vi "RGB_panicle_processing.vi"() -> ()   [LabVIEW 2019]
uses:
  <vilib>/Utility/file.llb/Read Delimited Spreadsheet (string).vi
  <vilib>/Utility/file.llb/Write Delimited Spreadsheet (string).vi
  <vilib>/vision/NI_Vision_Development_Module.lvlib
  <vilib>/Analysis/NI_AALBase.lvlib
  imFillRemove_vs2019/x64/Release/imFillRemove_vs2019.dll
panel:
  out "mean":dbl format="%0.2f"
  out "sum":dbl
  in  "图片存储":path=path "I:/rice_panicle/org/segment"
  out "Combine Image 7":T1(plugin-control)
  in  "图片来源":path=path "I:/rice_panicle/org/barcode1.txt"
  out "standard deviation 9":dbl format="%0.2f"
  out "mean 9":dbl format="%0.2f"
  out "standard deviation 8":dbl format="%0.2f"
  out "mean 8":dbl format="%0.2f"
  out "standard deviation 7":dbl format="%0.2f"
  out "mean 7":dbl format="%0.2f"
  out "standard deviation 6":dbl format="%0.2f"
  out "mean 6":dbl format="%0.2f"
  out "standard deviation 5":dbl format="%0.2f"
  out "mean 5":dbl format="%0.2f"
  out "Circularity":dbl[](array[numeric])
  out "Equivalent ellipse":dbl[](array[numeric])
  out "AR":dbl[](array[numeric])
  out "Perimeter":dbl[](array[numeric])
  out "Area":dbl[](array[numeric])
  out "耗时":u32
  out "属于某个角度下图像":T1(plugin-control)
  out "粒长":dbl[](array[numeric])
  out "粒宽":dbl[](array[numeric])
  out "长宽比":dbl[](array[numeric])
  out "mean 2":dbl format="%0.2f"
  out "standard deviation 2":dbl format="%0.2f"
  out "mean 3":dbl format="%0.2f"
  out "standard deviation 3":dbl format="%0.2f"
  out "mean 4":dbl format="%0.2f"
  out "standard deviation 4":dbl format="%0.2f"
  in  "数据存储":path=path "I:/rice_panicle/org/data.txt"
  out "估算粒子数目":dbl
  out "Combine Image 6":T1(plugin-control)
  out "selected path":path
  out "Combine Image 5":T1(plugin-control)
  out "Combine Image 4":T1(plugin-control)
  out "Combine Image 3":T1(plugin-control)
  out "Combine Image 2":T1(plugin-control)
  out "Combine Image":T1(plugin-control)
  in  "Range Upper Value":dbl=1200.0
  in  "Range Lower Value":dbl=600.0
  out "Number of Particles 2":i32
  in  "Removeareathreshold 3":i32=600
  in  "Range":cluster{"Lower value":sgl, "Upper value":sgl}={"Lower value"=0.0, "Upper value"=128.0}
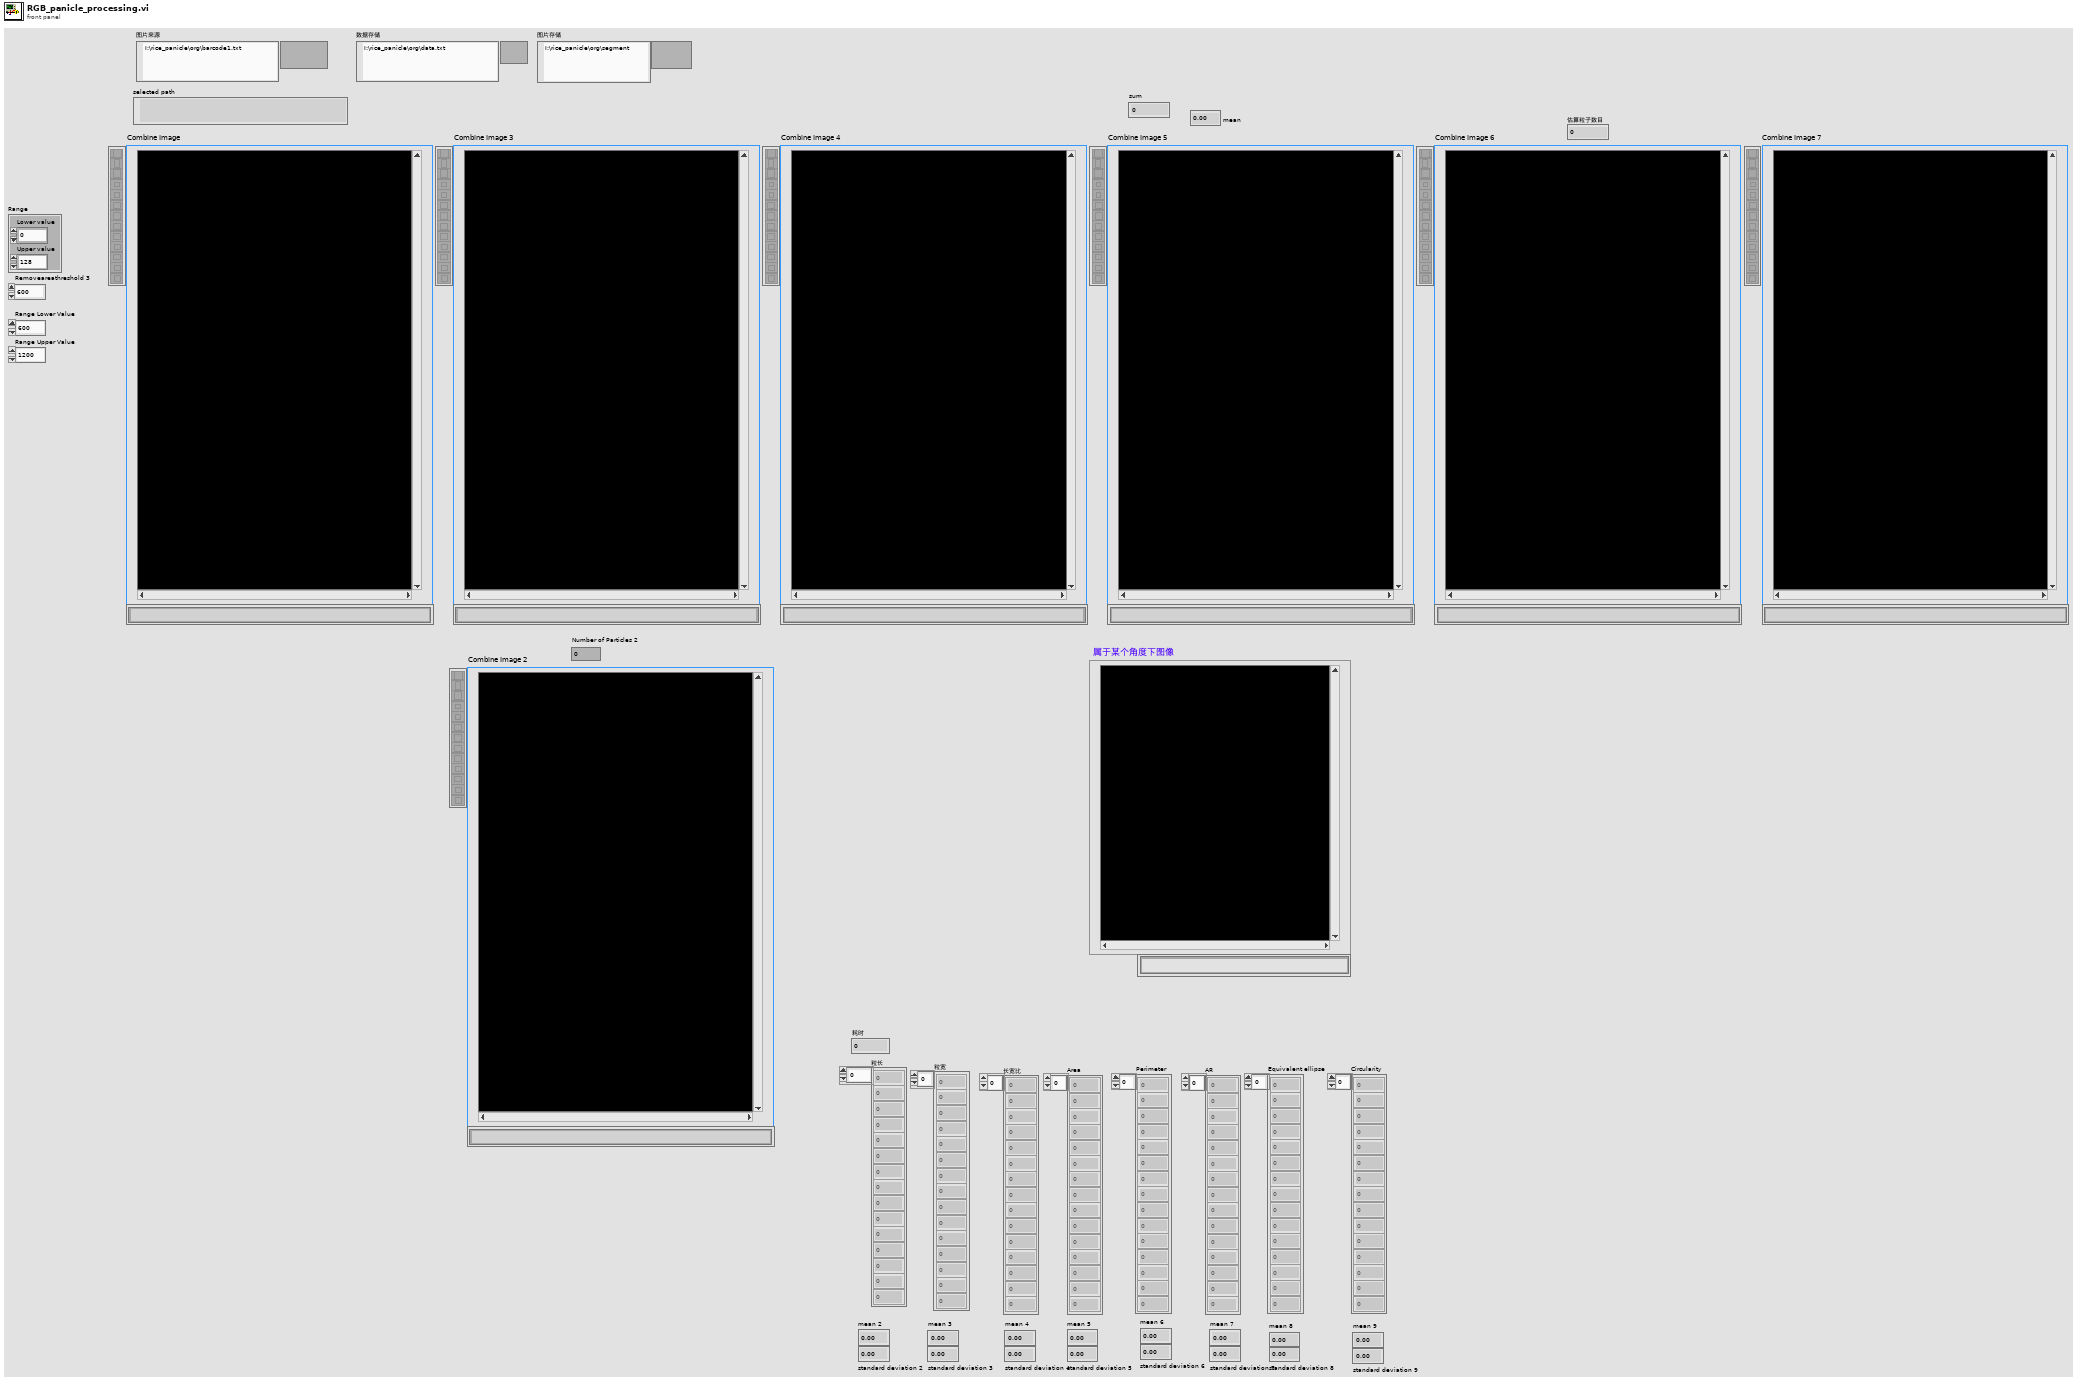
[diagram p1: front panel]
types:
  T1 = typedef "IMAQ Image.ctl" = refnum<image>
  T2 = typedef "Particle Parameters" = i32
  T3 = cluster{"Measurement Parameter":T2, "Range Lower Value":dbl, "Range Upper Value":dbl, "Range":bool, "Measurement Type":bool}
  T4 = enum32{"AutoM", "Close", "Dilate", "Erode", "Gradient", "Gradient out", "Gradient in", "Hit miss", "Open", "PClose", "POpen", "Thick", "Thin"}
  T5 = typedef "Image Type" = u32
  T6 = cluster{"Measurement Parameter":T2, "Range Lower Value":dbl, "Range Upper Value":dbl, "Range":bool, "Measurement Type":bool}[]
  T7 = cluster{"Measurement Parameter":T2, dbl, dbl, "Range":bool, "Measurement Type":bool}
  T8 = cluster{"Measurement Parameter":T2, dbl, dbl, "Range":bool, "Measurement Type":bool}[]
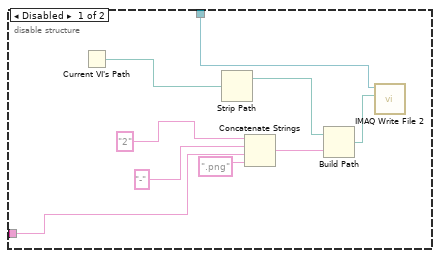
[diagram p2: hidden frame]
diagram:
  n1 = call-poly <vilib>:"Read Delimited Spreadsheet.vi"("file path (dialog if empty)"="图片来源") -> ("all rows"=w4:string[][])  [unwired: 9 in, 5 out]
  n2 = Index Array(array=w4, index (col)=0 ("disabled index (col)")) -> (element=w2:string[])  [unwired: 1 in]
  n3 = for {
    N: 1516 -> [_]
    tunnel: w2 -> [w46] mode=indexing
    w15 = T5 0 items=["Grayscale (U8)", "Grayscale (I16)", "Grayscale (SGL)", "Complex (CSG)", "RGB (U32)", "HSL (U32)", "RGB (U64)", "Grayscale (U16)"] ("Image Type")
    w22 = T5 0 items=["Grayscale (U8)", "Grayscale (I16)", "Grayscale (SGL)", "Complex (CSG)", "RGB (U32)", "HSL (U32)", "RGB (U64)", "Grayscale (U16)"] ("Image Type")
    w34 = T5 4 items=["Grayscale (U8)", "Grayscale (I16)", "Grayscale (SGL)", "Complex (CSG)", "RGB (U32)", "HSL (U32)", "RGB (U64)", "Grayscale (U16)"] ("Image Type")
    w79 = T2[] [35, 19, 32, 50, 55] items=["Center of Mass X", "Center of Mass Y", "First Pixel X", "First Pixel Y", "Bounding Rect Left", "Bounding Rect Top", "Bounding Rect Right", "Bounding Rect Bottom", "Max Feret Diameter Start X", "Max Feret Diameter Start Y", "Max Feret Diameter End X", "Max Feret Diameter End Y", "Max Horiz. Segment Length Left", "Max Horiz. Segment Length Right", "Max Horiz. Segment Length Row", "-", "Bounding Rect Width", "Bounding Rect Height", "Bounding Rect Diagonal", "Perimeter", "Convex Hull Perimeter", "Holes' Perimeter", "Max Feret Diameter", "Equivalent Ellipse Major Axis", "Equivalent Ellipse Minor Axis", "Equivalent Ellipse Minor Axis (Feret)", "Equivalent Rect Long Side", "Equivalent Rect Short Side", "Equivalent Rect Diagonal", "Equivalent Rect Short Side (Feret)", "Average Horiz. Segment Length", "Average Vert. Segment Length", "Hydraulic Radius", "Waddel Disk Diameter", "-", "Area", "Holes' Area", "Particle & Holes' Area", "Convex Hull Area", "Image Area", "-", "Number of Holes", "Number of Horiz. Segments", "Number of Vert. Segments", "-", "Orientation", "Max Feret Diameter Orientation", "-", "% Area/Image Area", "% Area/(Particle & Holes' Area)", "Ratio of Equivalent Ellipse Axes", "Ratio of Equivalent Rect Sides", "-", "Elongation Factor", "Compactness Factor", "Heywood Circularity Factor", "Type Factor", "-", "Sum X", "Sum Y", "Sum XX", "Sum XY", "Sum YY", "Sum XXX", "Sum XXY", "Sum XYY", "Sum YYY", "-", "Moment of Inertia XX", "Moment of Inertia XY", "Moment of Inertia YY", "Moment of Inertia XXX", "Moment of Inertia XXY", "Moment of Inertia XYY", "Moment of Inertia YYY", "Norm. Moment of Inertia XX", "Norm. Moment of Inertia XY", "Norm. Moment of Inertia YY", "Norm. Moment of Inertia XXX", "Norm. Moment of Inertia XXY", "Norm. Moment of Inertia XYY", "Norm. Moment of Inertia YYY", "Hu Moment 1", "Hu Moment 2", "Hu Moment 3", "Hu Moment 4", "Hu Moment 5", "Hu Moment 6", "Hu Moment 7"] ("Pixel Measurements")
    w88 = T2[] [35] items=["Center of Mass X", "Center of Mass Y", "First Pixel X", "First Pixel Y", "Bounding Rect Left", "Bounding Rect Top", "Bounding Rect Right", "Bounding Rect Bottom", "Max Feret Diameter Start X", "Max Feret Diameter Start Y", "Max Feret Diameter End X", "Max Feret Diameter End Y", "Max Horiz. Segment Length Left", "Max Horiz. Segment Length Right", "Max Horiz. Segment Length Row", "-", "Bounding Rect Width", "Bounding Rect Height", "Bounding Rect Diagonal", "Perimeter", "Convex Hull Perimeter", "Holes' Perimeter", "Max Feret Diameter", "Equivalent Ellipse Major Axis", "Equivalent Ellipse Minor Axis", "Equivalent Ellipse Minor Axis (Feret)", "Equivalent Rect Long Side", "Equivalent Rect Short Side", "Equivalent Rect Diagonal", "Equivalent Rect Short Side (Feret)", "Average Horiz. Segment Length", "Average Vert. Segment Length", "Hydraulic Radius", "Waddel Disk Diameter", "-", "Area", "Holes' Area", "Particle & Holes' Area", "Convex Hull Area", "Image Area", "-", "Number of Holes", "Number of Horiz. Segments", "Number of Vert. Segments", "-", "Orientation", "Max Feret Diameter Orientation", "-", "% Area/Image Area", "% Area/(Particle & Holes' Area)", "Ratio of Equivalent Ellipse Axes", "Ratio of Equivalent Rect Sides", "-", "Elongation Factor", "Compactness Factor", "Heywood Circularity Factor", "Type Factor", "-", "Sum X", "Sum Y", "Sum XX", "Sum XY", "Sum YY", "Sum XXX", "Sum XXY", "Sum XYY", "Sum YYY", "-", "Moment of Inertia XX", "Moment of Inertia XY", "Moment of Inertia YY", "Moment of Inertia XXX", "Moment of Inertia XXY", "Moment of Inertia XYY", "Moment of Inertia YYY", "Norm. Moment of Inertia XX", "Norm. Moment of Inertia XY", "Norm. Moment of Inertia YY", "Norm. Moment of Inertia XXX", "Norm. Moment of Inertia XXY", "Norm. Moment of Inertia XYY", "Norm. Moment of Inertia YYY", "Hu Moment 1", "Hu Moment 2", "Hu Moment 3", "Hu Moment 4", "Hu Moment 5", "Hu Moment 6", "Hu Moment 7"] ("Pixel Measurements")
    w92 = T2[] [35] items=["Center of Mass X", "Center of Mass Y", "First Pixel X", "First Pixel Y", "Bounding Rect Left", "Bounding Rect Top", "Bounding Rect Right", "Bounding Rect Bottom", "Max Feret Diameter Start X", "Max Feret Diameter Start Y", "Max Feret Diameter End X", "Max Feret Diameter End Y", "Max Horiz. Segment Length Left", "Max Horiz. Segment Length Right", "Max Horiz. Segment Length Row", "-", "Bounding Rect Width", "Bounding Rect Height", "Bounding Rect Diagonal", "Perimeter", "Convex Hull Perimeter", "Holes' Perimeter", "Max Feret Diameter", "Equivalent Ellipse Major Axis", "Equivalent Ellipse Minor Axis", "Equivalent Ellipse Minor Axis (Feret)", "Equivalent Rect Long Side", "Equivalent Rect Short Side", "Equivalent Rect Diagonal", "Equivalent Rect Short Side (Feret)", "Average Horiz. Segment Length", "Average Vert. Segment Length", "Hydraulic Radius", "Waddel Disk Diameter", "-", "Area", "Holes' Area", "Particle & Holes' Area", "Convex Hull Area", "Image Area", "-", "Number of Holes", "Number of Horiz. Segments", "Number of Vert. Segments", "-", "Orientation", "Max Feret Diameter Orientation", "-", "% Area/Image Area", "% Area/(Particle & Holes' Area)", "Ratio of Equivalent Ellipse Axes", "Ratio of Equivalent Rect Sides", "-", "Elongation Factor", "Compactness Factor", "Heywood Circularity Factor", "Type Factor", "-", "Sum X", "Sum Y", "Sum XX", "Sum XY", "Sum YY", "Sum XXX", "Sum XXY", "Sum XYY", "Sum YYY", "-", "Moment of Inertia XX", "Moment of Inertia XY", "Moment of Inertia YY", "Moment of Inertia XXX", "Moment of Inertia XXY", "Moment of Inertia XYY", "Moment of Inertia YYY", "Norm. Moment of Inertia XX", "Norm. Moment of Inertia XY", "Norm. Moment of Inertia YY", "Norm. Moment of Inertia XXX", "Norm. Moment of Inertia XXY", "Norm. Moment of Inertia XYY", "Norm. Moment of Inertia YYY", "Hu Moment 1", "Hu Moment 2", "Hu Moment 3", "Hu Moment 4", "Hu Moment 5", "Hu Moment 6", "Hu Moment 7"] ("Pixel Measurements")
    w100 = T5 0 items=["Grayscale (U8)", "Grayscale (I16)", "Grayscale (SGL)", "Complex (CSG)", "RGB (U32)", "HSL (U32)", "RGB (U64)", "Grayscale (U16)"] ("Image Type")
    w107 = T5 0 items=["Grayscale (U8)", "Grayscale (I16)", "Grayscale (SGL)", "Complex (CSG)", "RGB (U32)", "HSL (U32)", "RGB (U64)", "Grayscale (U16)"] ("Image Type")
    w121 = T5 0 items=["Grayscale (U8)", "Grayscale (I16)", "Grayscale (SGL)", "Complex (CSG)", "RGB (U32)", "HSL (U32)", "RGB (U64)", "Grayscale (U16)"] ("Image Type")
    w126 = T5 0 items=["Grayscale (U8)", "Grayscale (I16)", "Grayscale (SGL)", "Complex (CSG)", "RGB (U32)", "HSL (U32)", "RGB (U64)", "Grayscale (U16)"] ("Image Type")
    w131 = T5 0 items=["Grayscale (U8)", "Grayscale (I16)", "Grayscale (SGL)", "Complex (CSG)", "RGB (U32)", "HSL (U32)", "RGB (U64)", "Grayscale (U16)"] ("Image Type")
    w135 = T5 0 items=["Grayscale (U8)", "Grayscale (I16)", "Grayscale (SGL)", "Complex (CSG)", "RGB (U32)", "HSL (U32)", "RGB (U64)", "Grayscale (U16)"] ("Image Type")
    w148 = T5 0 items=["Grayscale (U8)", "Grayscale (I16)", "Grayscale (SGL)", "Complex (CSG)", "RGB (U32)", "HSL (U32)", "RGB (U64)", "Grayscale (U16)"] ("Image Type")
    w166 = 0 items=["Red", "Green", "Blue", "Hue", "Saturation", "Luminance", "Value", "Intensity"] ("Color Plane")
    w167 = T5 4 items=["Grayscale (U8)", "Grayscale (I16)", "Grayscale (SGL)", "Complex (CSG)", "RGB (U32)", "HSL (U32)", "RGB (U64)", "Grayscale (U16)"] ("Image Type")
    # "有些主茎可能还是去不掉，必须用面积阈值去除"
    # "挑选出不粘连的粒子做下一步处理"
    # "去掉标签纸"
    # "去掉主茎"
    # "去除小区域"
    n4 = String To Path(string=w46) -> (path=w42:path)
    "selected path" <- w42
    n5 = Path To String(path=w42) -> (string=w41:string)
    n6 = Reverse String(1:w41) -> (0:w44:string)
    n7 = call "IMAQ Create"("Image Name"="untitled", "Image Type"=w167) -> ("New Image"=w169:T1, "error out"=w168:errorcluster)  [unwired: 2 in, 1 out]
    n8 = Search/Split String(string=w44, search string/char (-)="\\" ("pattern")) -> (substring before match=w45:string)  [unwired: 3 out]
    n9 = call "IMAQ ReadFile"("File Path"=w42, "error in (no error)"=w168, "Image"=w169) -> ("error out"=w170:errorcluster, "Image Out"=w36:T1)  [unwired: 2 in, 5 out]
    "Combine Image" <- w36
    n10 = Reverse String(1:w45) -> (0:w40:string)
    n11 = String Subset(string=w40, length (rest)=6 ("length (rest)")) -> (substring=w25:string)  [unwired: 1 in]
    n12 = call "IMAQ Create"("Image Name"="S0", "Image Type"=w131) -> ("New Image"=w129:T1)  [unwired: 2 in, 2 out]
    n13 = call "IMAQ ExtractSingleColorPlane"("Color Plane"=w166, "error in (no error)"=w170, "Image Dst"=w129, "Image Src"=w36) -> ("error out"=w165:errorcluster, "Image Dst Out"=w163:T1)  [unwired: 6 out]
    n14 = call "IMAQ Threshold"("error in (no error)"=w165, "Range"="Range", "Image Src"=w163) -> ("error out"=w162:errorcluster, "Image Dst Out"=w157:T1)  [unwired: 3 in, 4 out]
    n15 = call "IMAQ Morphology"("Number of iterations (1)"=2, "Structuring Element"=i32[][] [[0, 1, 0], [1, 1, 1], [0, 1, 0]], "Square/Hexa (Square)"=FALSE, "error in (no error)"=w162, "Operation"=T4."Erode", "Image Src"=w157) -> ("error out"=w156:errorcluster, "Image Dst Out"=w151:T1)  [unwired: 1 in, 3 out]
    n16 = call "IMAQ Morphology"("Number of iterations (1)"=2, "Structuring Element"=i32[][] [[0, 1, 0], [1, 1, 1], [0, 1, 0]], "Square/Hexa (Square)"=FALSE, "error in (no error)"=w156, "Operation"=T4."Dilate", "Image Src"=w151) -> ("Image Dst Out"=w142:T1)  [unwired: 1 in, 4 out]
    n17 = call "IMAQ ImageToArray"("Image"=w142) -> ("Image Pixels (U8)"=w143:u8[][])  [unwired: 2 in, 5 out]
    n18 = call "IMAQ GetImageSize"("Image"=w142) -> ("Y Resolution"=w145:i32, "X Resolution"=w144:i32)  [unwired: 1 in, 3 out]
    n19 = call "IMAQ Create"("Image Name"="S1", "Image Type"=w148) -> ("New Image"=w146:T1)  [unwired: 2 in, 2 out]
    n20 = dll-call lib="G:/preprocessing/rice_panicle/imFillRemove_vs2019/x64/Release/imFillRemove_vs2019.dll" fn="bwremove"("bw"=w143, "row"=w145, "col"=w144, "areathreshold"="Removeareathreshold 3") -> ("bw"=w150:u8[][])  [unwired: 6 in, 3 out]
    n21 = call "IMAQ ArrayToImage"("Image Pixels (U8)"=w150, "Image"=w146) -> ("Image Out"=w128:T1)  [unwired: 4 in, 5 out]
    n22 = call "IMAQ Create"("Image Name"="S2", "Image Type"=w126) -> ("New Image"=w125:T1)  [unwired: 2 in, 2 out]
    n23 = call "IMAQ RejectBorder"("Image Dst"=w125, "Image Src"=w128) -> ("Image Dst Out"=w114:T1)  [unwired: 4 in, 1 out]
    "Combine Image 3" <- w114
    n24 = Bundle(cluster=T3 {"Measurement Parameter"=35, "Range Lower Value"=0.0, "Range Upper Value"=0.0, "Range"=FALSE, "Measurement Type"=FALSE} ("Selection Value"), "Range Lower Value"="Range Lower Value", "Range Upper Value"="Range Upper Value") -> (w139:T3)  [unwired: 3 out]
    n25 = Initialize Array(w139, 1 ("dimension size")) -> (w140:T6)
    n26 = call "IMAQ Create"("Image Name"="S3", "Image Type"=w135) -> ("New Image"=w137:T1)  [unwired: 2 in, 2 out]
    n27 = call "IMAQ Particle Filter 3"("Image Src"=w114, "Image Dst"=w137, "Selection Values"=w140, "Keep/Remove Particles (F)"=FALSE) -> ("Image Dst Out"=w8:T1)  [unwired: 5 in, 6 out]
    n28 = Bundle(cluster=T3 {"Measurement Parameter"=53, "Range Lower Value"=0.0, "Range Upper Value"=0.0, "Range"=FALSE, "Measurement Type"=FALSE} ("Selection Value"), "Range Lower Value"=0.0 ("Range Lower Value 2"), "Range Upper Value"=15.0 ("Range Upper Value 2")) -> (w117:T3)  [unwired: 3 out]
    n29 = Initialize Array(w117, 1 ("dimension size")) -> (w116:T6)
    n30 = call "IMAQ Create"("Image Name"="S4", "Image Type"=w121) -> ("New Image"=w119:T1)  [unwired: 2 in, 2 out]
    n31 = call "IMAQ Particle Filter 3"("Image Src"=w114, "Image Dst"=w119, "Selection Values"=w116, "Keep/Remove Particles (F)"=FALSE) -> ("Image Dst Out"=w103:T1)  [unwired: 5 in, 6 out]
    "Combine Image 4" <- w103
    n32 = Bundle(cluster=T3 {"Measurement Parameter"=53, "Range Lower Value"=0.0, "Range Upper Value"=0.0, "Range"=FALSE, "Measurement Type"=FALSE} ("Selection Value"), "Range Lower Value"=0.0 ("Range Lower Value 2"), "Range Upper Value"=15.0 ("Range Upper Value 2")) -> (w11:T3)  [unwired: 3 out]
    n33 = Initialize Array(w11, 1 ("dimension size")) -> (w10:T6)
    n34 = call "IMAQ Create"("Image Name"="S10", "Image Type"=w15) -> ("New Image"=w13:T1)  [unwired: 2 in, 2 out]
    n35 = call "IMAQ Particle Filter 3"("Image Src"=w8, "Image Dst"=w13, "Selection Values"=w10, "Keep/Remove Particles (F)"=FALSE) -> ("Image Dst Out"=w6:T1, "Number of Particles"=w7:i32)  [unwired: 5 in, 5 out]
    "Number of Particles 2" <- w7
    "Combine Image 2" <- w6
    n36 = Bundle(cluster=T3 {"Measurement Parameter"=41, "Range Lower Value"=0.0, "Range Upper Value"=0.0, "Range"=FALSE, "Measurement Type"=FALSE} ("Selection Value"), "Range Lower Value"=6.0 ("Range Lower Value 2"), "Range Upper Value"=10000.0 ("Range Upper Value 2")) -> (w111:T3)  [unwired: 3 out]
    n37 = Initialize Array(w111, 1 ("dimension size")) -> (w112:T6)
    n38 = call "IMAQ Create"("Image Name"="S5", "Image Type"=w107) -> ("New Image"=w109:T1)  [unwired: 2 in, 2 out]
    n39 = call "IMAQ Particle Filter 3"("Image Src"=w103, "Image Dst"=w109, "Selection Values"=w112, "Keep/Remove Particles (F)"=TRUE) -> ("Image Dst Out"=w93:T1)  [unwired: 5 in, 6 out]
    "Combine Image 5" <- w93
    n40 = call "IMAQ Particle Analysis"("Pixel Measurements"=w92, "Image"=w6) -> ("Particle Measurements (Pixels)"=w90:dbl[][])  [unwired: 3 in, 6 out]
    n41 = Index Array(array=w90, index (col)=0 ("index (row)")) -> (element=w89:dbl[])  [unwired: 1 in]
    n42 = call <vilib>:"Std Deviation and Variance.vi"("X"=w89) -> ("mean"=w85:dbl)  [unwired: 1 in, 2 out]
    "mean" <- w85
    n43 = Bundle(cluster=T3 {"Measurement Parameter"=35, "Range Lower Value"=0.0, "Range Upper Value"=0.0, "Range"=FALSE, "Measurement Type"=FALSE} ("Selection Value"), "Range Lower Value"=8000.0 ("Range Lower Value 2")) -> (w96:T3)  [unwired: 4 out]
    n44 = Initialize Array(w96, 1 ("dimension size")) -> (w95:T6)
    n45 = call "IMAQ Create"("Image Name"="S6", "Image Type"=w100) -> ("New Image"=w98:T1)  [unwired: 2 in, 2 out]
    n46 = call "IMAQ Particle Filter 3"("Image Src"=w93, "Image Dst"=w98, "Selection Values"=w95, "Keep/Remove Particles (F)"=TRUE) -> ("Image Dst Out"=w37:T1)  [unwired: 5 in, 6 out]
    "Combine Image 6" <- w37
    n47 = call "IMAQ Create"("Image Name"="save1", "Image Type"=w22) -> ("New Image"=w19:T1, "error out"=w20:errorcluster)  [unwired: 2 in, 1 out]
    n48 = call <vilib>:"IVA Binary Inverse.vi"("error in (no error)"=w20, "Image In"=w37) -> ("Image Out"=w32:T1)  [unwired: 9 out]
    n49 = call "IMAQ Multiply"("Image Src A"=w32, "Constant"=255.0, "Image Dst"=w19) -> ("Image Dst Out"=w30:T1)  [unwired: 4 in, 1 out]
    n50 = call "IMAQ Particle Analysis"("Pixel Measurements"=w88, "Image"=w37) -> ("Particle Measurements (Pixels)"=w86:dbl[][])  [unwired: 3 in, 6 out]
    n51 = Index Array(array=w86, index (col)=0 ("index (row)")) -> (element=w84:dbl[])  [unwired: 1 in]
    n52 = Add Array Elements(numeric array=w84) -> (sum=w83:dbl)
    "sum" <- w83
    n53 = call "IMAQ Create"("Image Name"="save", "Image Type"=w34) -> ("New Image"=w33:T1)  [unwired: 2 in, 2 out]
    n54 = Divide(x=w83, y=w85) -> (x/y=w49:dbl)
    "估算粒子数目" <- w49
    n55 = To Long Integer(number=w49) -> (32bit integer=w48:i32)
    n56 = Number To Decimal String(number=w48) -> (decimal integer string=w47:string)  [unwired: 1 in]
    n57 = call "IMAQ Add"("Image Src A"=w36, "Image Dst"=w33, "Image Src B"=w30) -> ("Image Dst Out"=w24:T1)  [unwired: 4 in, 1 out]
    "Combine Image 7" <- w24
    n58 = flat-sequence {
      tunnel: w7 -> [w182]
      tunnel: w6 -> [w183]
      tunnel: [w183] -> w180
      tunnel: [w182] -> w179
      tunnel: [w181] -> w178
      tunnel: w180 -> [w199]
      tunnel: w179 -> [w198]
      tunnel: w178 -> [w197]
      tunnel: [w197] -> w177
      tunnel: [w189] -> w176
      tunnel: [w188] -> w175
      tunnel: [w187] -> w174
      tunnel: [w186] -> w173
      tunnel: [w185] -> w172
      tunnel: [w184] -> w171
      tunnel: w177 -> [w279]
      tunnel: [w277] -> w67
      tunnel: w176 -> [w277]
      tunnel: [w276] -> w66
      tunnel: w175 -> [w276]
      tunnel: [w275] -> w65
      tunnel: w174 -> [w275]
      tunnel: [w274] -> w64
      tunnel: w173 -> [w274]
      tunnel: [w273] -> w63
      tunnel: w172 -> [w273]
      tunnel: [w272] -> w62
      tunnel: w171 -> [w272]
      frame #0 {
        n59 = Tick Count (ms)() -> (millisecond timer value=w181:u32)
      }
      frame #1 {
        w208 = T2[] [0, 1, 45] items=["Center of Mass X", "Center of Mass Y", "First Pixel X", "First Pixel Y", "Bounding Rect Left", "Bounding Rect Top", "Bounding Rect Right", "Bounding Rect Bottom", "Max Feret Diameter Start X", "Max Feret Diameter Start Y", "Max Feret Diameter End X", "Max Feret Diameter End Y", "Max Horiz. Segment Length Left", "Max Horiz. Segment Length Right", "Max Horiz. Segment Length Row", "-", "Bounding Rect Width", "Bounding Rect Height", "Bounding Rect Diagonal", "Perimeter", "Convex Hull Perimeter", "Holes' Perimeter", "Max Feret Diameter", "Equivalent Ellipse Major Axis", "Equivalent Ellipse Minor Axis", "Equivalent Ellipse Minor Axis (Feret)", "Equivalent Rect Long Side", "Equivalent Rect Short Side", "Equivalent Rect Diagonal", "Equivalent Rect Short Side (Feret)", "Average Horiz. Segment Length", "Average Vert. Segment Length", "Hydraulic Radius", "Waddel Disk Diameter", "-", "Area", "Holes' Area", "Particle & Holes' Area", "Convex Hull Area", "Image Area", "-", "Number of Holes", "Number of Horiz. Segments", "Number of Vert. Segments", "-", "Orientation", "Max Feret Diameter Orientation", "-", "% Area/Image Area", "% Area/(Particle & Holes' Area)", "Ratio of Equivalent Ellipse Axes", "Ratio of Equivalent Rect Sides", "-", "Elongation Factor", "Compactness Factor", "Heywood Circularity Factor", "Type Factor", "-", "Sum X", "Sum Y", "Sum XX", "Sum XY", "Sum YY", "Sum XXX", "Sum XXY", "Sum XYY", "Sum YYY", "-", "Moment of Inertia XX", "Moment of Inertia XY", "Moment of Inertia YY", "Moment of Inertia XXX", "Moment of Inertia XXY", "Moment of Inertia XYY", "Moment of Inertia YYY", "Norm. Moment of Inertia XX", "Norm. Moment of Inertia XY", "Norm. Moment of Inertia YY", "Norm. Moment of Inertia XXX", "Norm. Moment of Inertia XXY", "Norm. Moment of Inertia XYY", "Norm. Moment of Inertia YYY", "Hu Moment 1", "Hu Moment 2", "Hu Moment 3", "Hu Moment 4", "Hu Moment 5", "Hu Moment 6", "Hu Moment 7"] ("Pixel Measurements")
        # "粒宽"
        # "粒长"
        n60 = call "IMAQ Particle Analysis"("Pixel Measurements"=w208, "Image"=w199) -> ("Particle Measurements (Pixels)"=w206:dbl[][], "Image Out (duplicate)"=w207:T1)  [unwired: 3 in, 5 out]
        n61 = Index Array(array=w206, index (col) #1=0 ("disabled index (col)"), index (col) #2=1 ("index (col)"), index (col) #3=2 ("index (col)")) -> (element #1=w202:dbl[], element #2=w201:dbl[], element #3=w200:dbl[])  [unwired: 3 in]
        n62 = for {
          N: w198 -> [_]
          tunnel: w207 -> [w260]
          tunnel: w202 -> [w237] mode=indexing
          tunnel: w201 -> [w231] mode=indexing
          tunnel: w200 -> [w252] mode=indexing
          tunnel: [w243] -> _ mode=indexing
          tunnel: [w220] -> w193 mode=indexing
          tunnel: [w217] -> w194 mode=indexing
          i -> [w249]
          w218 = T2[] [17] items=["Center of Mass X", "Center of Mass Y", "First Pixel X", "First Pixel Y", "Bounding Rect Left", "Bounding Rect Top", "Bounding Rect Right", "Bounding Rect Bottom", "Max Feret Diameter Start X", "Max Feret Diameter Start Y", "Max Feret Diameter End X", "Max Feret Diameter End Y", "Max Horiz. Segment Length Left", "Max Horiz. Segment Length Right", "Max Horiz. Segment Length Row", "-", "Bounding Rect Width", "Bounding Rect Height", "Bounding Rect Diagonal", "Perimeter", "Convex Hull Perimeter", "Holes' Perimeter", "Max Feret Diameter", "Equivalent Ellipse Major Axis", "Equivalent Ellipse Minor Axis", "Equivalent Ellipse Minor Axis (Feret)", "Equivalent Rect Long Side", "Equivalent Rect Short Side", "Equivalent Rect Diagonal", "Equivalent Rect Short Side (Feret)", "Average Horiz. Segment Length", "Average Vert. Segment Length", "Hydraulic Radius", "Waddel Disk Diameter", "-", "Area", "Holes' Area", "Particle & Holes' Area", "Convex Hull Area", "Image Area", "-", "Number of Holes", "Number of Horiz. Segments", "Number of Vert. Segments", "-", "Orientation", "Max Feret Diameter Orientation", "-", "% Area/Image Area", "% Area/(Particle & Holes' Area)", "Ratio of Equivalent Ellipse Axes", "Ratio of Equivalent Rect Sides", "-", "Elongation Factor", "Compactness Factor", "Heywood Circularity Factor", "Type Factor", "-", "Sum X", "Sum Y", "Sum XX", "Sum XY", "Sum YY", "Sum XXX", "Sum XXY", "Sum XYY", "Sum YYY", "-", "Moment of Inertia XX", "Moment of Inertia XY", "Moment of Inertia YY", "Moment of Inertia XXX", "Moment of Inertia XXY", "Moment of Inertia XYY", "Moment of Inertia YYY", "Norm. Moment of Inertia XX", "Norm. Moment of Inertia XY", "Norm. Moment of Inertia YY", "Norm. Moment of Inertia XXX", "Norm. Moment of Inertia XXY", "Norm. Moment of Inertia XYY", "Norm. Moment of Inertia YYY", "Hu Moment 1", "Hu Moment 2", "Hu Moment 3", "Hu Moment 4", "Hu Moment 5", "Hu Moment 6", "Hu Moment 7"] ("Pixel Measurements")
          w223 = T2[] [16] items=["Center of Mass X", "Center of Mass Y", "First Pixel X", "First Pixel Y", "Bounding Rect Left", "Bounding Rect Top", "Bounding Rect Right", "Bounding Rect Bottom", "Max Feret Diameter Start X", "Max Feret Diameter Start Y", "Max Feret Diameter End X", "Max Feret Diameter End Y", "Max Horiz. Segment Length Left", "Max Horiz. Segment Length Right", "Max Horiz. Segment Length Row", "-", "Bounding Rect Width", "Bounding Rect Height", "Bounding Rect Diagonal", "Perimeter", "Convex Hull Perimeter", "Holes' Perimeter", "Max Feret Diameter", "Equivalent Ellipse Major Axis", "Equivalent Ellipse Minor Axis", "Equivalent Ellipse Minor Axis (Feret)", "Equivalent Rect Long Side", "Equivalent Rect Short Side", "Equivalent Rect Diagonal", "Equivalent Rect Short Side (Feret)", "Average Horiz. Segment Length", "Average Vert. Segment Length", "Hydraulic Radius", "Waddel Disk Diameter", "-", "Area", "Holes' Area", "Particle & Holes' Area", "Convex Hull Area", "Image Area", "-", "Number of Holes", "Number of Horiz. Segments", "Number of Vert. Segments", "-", "Orientation", "Max Feret Diameter Orientation", "-", "% Area/Image Area", "% Area/(Particle & Holes' Area)", "Ratio of Equivalent Ellipse Axes", "Ratio of Equivalent Rect Sides", "-", "Elongation Factor", "Compactness Factor", "Heywood Circularity Factor", "Type Factor", "-", "Sum X", "Sum Y", "Sum XX", "Sum XY", "Sum YY", "Sum XXX", "Sum XXY", "Sum XYY", "Sum YYY", "-", "Moment of Inertia XX", "Moment of Inertia XY", "Moment of Inertia YY", "Moment of Inertia XXX", "Moment of Inertia XXY", "Moment of Inertia XYY", "Moment of Inertia YYY", "Norm. Moment of Inertia XX", "Norm. Moment of Inertia XY", "Norm. Moment of Inertia YY", "Norm. Moment of Inertia XXX", "Norm. Moment of Inertia XXY", "Norm. Moment of Inertia XYY", "Norm. Moment of Inertia YYY", "Hu Moment 1", "Hu Moment 2", "Hu Moment 3", "Hu Moment 4", "Hu Moment 5", "Hu Moment 6", "Hu Moment 7"] ("Pixel Measurements")
          w226 = T5 0 items=["Grayscale (U8)", "Grayscale (I16)", "Grayscale (SGL)", "Complex (CSG)", "RGB (U32)", "HSL (U32)", "RGB (U64)", "Grayscale (U16)"] ("Image Type")
          w239 = T5 0 items=["Grayscale (U8)", "Grayscale (I16)", "Grayscale (SGL)", "Complex (CSG)", "RGB (U32)", "HSL (U32)", "RGB (U64)", "Grayscale (U16)"] ("Image Type")
          w256 = T2 1 items=["Center of Mass X", "Center of Mass Y", "First Pixel X", "First Pixel Y", "Bounding Rect Left", "Bounding Rect Top", "Bounding Rect Right", "Bounding Rect Bottom", "Max Feret Diameter Start X", "Max Feret Diameter Start Y", "Max Feret Diameter End X", "Max Feret Diameter End Y", "Max Horiz. Segment Length Left", "Max Horiz. Segment Length Right", "Max Horiz. Segment Length Row", "-", "Bounding Rect Width", "Bounding Rect Height", "Bounding Rect Diagonal", "Perimeter", "Convex Hull Perimeter", "Holes' Perimeter", "Max Feret Diameter", "Equivalent Ellipse Major Axis", "Equivalent Ellipse Minor Axis", "Equivalent Ellipse Minor Axis (Feret)", "Equivalent Rect Long Side", "Equivalent Rect Short Side", "Equivalent Rect Diagonal", "Equivalent Rect Short Side (Feret)", "Average Horiz. Segment Length", "Average Vert. Segment Length", "Hydraulic Radius", "Waddel Disk Diameter", "-", "Area", "Holes' Area", "Particle & Holes' Area", "Convex Hull Area", "Image Area", "-", "Number of Holes", "Number of Horiz. Segments", "Number of Vert. Segments", "-", "Orientation", "Max Feret Diameter Orientation", "-", "% Area/Image Area", "% Area/(Particle & Holes' Area)", "Ratio of Equivalent Ellipse Axes", "Ratio of Equivalent Rect Sides", "-", "Elongation Factor", "Compactness Factor", "Heywood Circularity Factor", "Type Factor", "-", "Sum X", "Sum Y", "Sum XX", "Sum XY", "Sum YY", "Sum XXX", "Sum XXY", "Sum XYY", "Sum YYY", "-", "Moment of Inertia XX", "Moment of Inertia XY", "Moment of Inertia YY", "Moment of Inertia XXX", "Moment of Inertia XXY", "Moment of Inertia XYY", "Moment of Inertia YYY", "Norm. Moment of Inertia XX", "Norm. Moment of Inertia XY", "Norm. Moment of Inertia YY", "Norm. Moment of Inertia XXX", "Norm. Moment of Inertia XXY", "Norm. Moment of Inertia XYY", "Norm. Moment of Inertia YYY", "Hu Moment 1", "Hu Moment 2", "Hu Moment 3", "Hu Moment 4", "Hu Moment 5", "Hu Moment 6", "Hu Moment 7"] ("Measurement Parameter")
          w259 = T2 0 items=["Center of Mass X", "Center of Mass Y", "First Pixel X", "First Pixel Y", "Bounding Rect Left", "Bounding Rect Top", "Bounding Rect Right", "Bounding Rect Bottom", "Max Feret Diameter Start X", "Max Feret Diameter Start Y", "Max Feret Diameter End X", "Max Feret Diameter End Y", "Max Horiz. Segment Length Left", "Max Horiz. Segment Length Right", "Max Horiz. Segment Length Row", "-", "Bounding Rect Width", "Bounding Rect Height", "Bounding Rect Diagonal", "Perimeter", "Convex Hull Perimeter", "Holes' Perimeter", "Max Feret Diameter", "Equivalent Ellipse Major Axis", "Equivalent Ellipse Minor Axis", "Equivalent Ellipse Minor Axis (Feret)", "Equivalent Rect Long Side", "Equivalent Rect Short Side", "Equivalent Rect Diagonal", "Equivalent Rect Short Side (Feret)", "Average Horiz. Segment Length", "Average Vert. Segment Length", "Hydraulic Radius", "Waddel Disk Diameter", "-", "Area", "Holes' Area", "Particle & Holes' Area", "Convex Hull Area", "Image Area", "-", "Number of Holes", "Number of Horiz. Segments", "Number of Vert. Segments", "-", "Orientation", "Max Feret Diameter Orientation", "-", "% Area/Image Area", "% Area/(Particle & Holes' Area)", "Ratio of Equivalent Ellipse Axes", "Ratio of Equivalent Rect Sides", "-", "Elongation Factor", "Compactness Factor", "Heywood Circularity Factor", "Type Factor", "-", "Sum X", "Sum Y", "Sum XX", "Sum XY", "Sum YY", "Sum XXX", "Sum XXY", "Sum XYY", "Sum YYY", "-", "Moment of Inertia XX", "Moment of Inertia XY", "Moment of Inertia YY", "Moment of Inertia XXX", "Moment of Inertia XXY", "Moment of Inertia XYY", "Moment of Inertia YYY", "Norm. Moment of Inertia XX", "Norm. Moment of Inertia XY", "Norm. Moment of Inertia YY", "Norm. Moment of Inertia XXX", "Norm. Moment of Inertia XXY", "Norm. Moment of Inertia XYY", "Norm. Moment of Inertia YYY", "Hu Moment 1", "Hu Moment 2", "Hu Moment 3", "Hu Moment 4", "Hu Moment 5", "Hu Moment 6", "Hu Moment 7"] ("Measurement Parameter")
          w262 = T5 0 items=["Grayscale (U8)", "Grayscale (I16)", "Grayscale (SGL)", "Complex (CSG)", "RGB (U32)", "HSL (U32)", "RGB (U64)", "Grayscale (U16)"] ("Image Type")
          n63 = Add(x=w237, y=2.0) -> (x+y=w241:dbl)
          n64 = Subtract(x=w237, y=2.0) -> (x-y=w235:dbl)
          n65 = Bundle("Measurement Parameter"=w259, w235, w241, "Range"=FALSE, "Measurement Type"=FALSE) -> (w253:T7)  [unwired: 1 out]
          n66 = call "IMAQ Create"("Image Name"="17", "Image Type"=w239) -> ("New Image"=w238:T1)  [unwired: 2 in, 2 out]
          n67 = Add(x=w231, y=2.0) -> (x+y=w229:dbl)
          n68 = Subtract(x=w231, y=2.0) -> (x-y=w230:dbl)
          n69 = Bundle("Measurement Parameter"=w256, w230, w229, "Range"=FALSE, "Measurement Type"=FALSE) -> (w228:T7)  [unwired: 1 out]
          n70 = Build Array(w253) -> (w234:T8)
          n71 = Build Array(w228) -> (w227:T8)
          n72 = Number To Decimal String(number=w249) -> (decimal integer string=w248:string)  [unwired: 1 out]
          n73 = call "IMAQ Particle Filter 3"("Image Src"=w260, "Image Dst"=w238, "Selection Values"=w234, "Keep/Remove Particles (F)"=FALSE) -> ("Image Dst Out"=w246:T1)  [unwired: 5 in, 6 out]
          n74 = Subtract(x=180.0, y=w252) -> (x-y=w250:dbl)
          n75 = call "IMAQ Create"("Image Name"="16", "Image Type"=w262) -> ("New Image"=w244:T1)  [unwired: 2 in, 2 out]
          n76 = call "IMAQ Particle Filter 3"("Image Src"=w246, "Image Dst"=w244, "Selection Values"=w227, "Keep/Remove Particles (F)"=FALSE) -> ("Image Dst Out"=w221:T1, "Number of Particles"=w243:i32)  [unwired: 5 in, 5 out]
          n77 = call "IMAQ Create"("Image Name"="18", "Image Type"=w226) -> ("New Image"=w224:T1)  [unwired: 2 in, 2 out]
          n78 = call "IMAQ Rotate"("Maintain Size"=FALSE, "Angle (degrees)"=w250, "Image Dst"=w224, "Image Src"=w221) -> ("Image Dst Out"=w219:T1)  [unwired: 4 in, 3 out]
          "属于某个角度下图像" <- w219
          n79 = disable-structure shown="Enabled" {
            disable-tunnel: w248 -> [w271 _]
            disable-tunnel: w219 -> [w263 _]
            frame Disabled {
              n80 = Current VI's Path() -> (path=w264:path)
              n81 = Strip Path(path=w264) -> (stripped path=w267:path)  [unwired: 1 out]
              n82 = Concatenate Strings("2" ("string"), "-" ("string"), w271, ".png") -> (w268:string)
              n83 = Build Path(base path=w267, name or relative path=w268) -> (appended path=w266:path)
              n84 = call-poly "IMAQ Write File 2"("File Path"=w266, "Image"=w263) -> ()  [unwired: 4 in, 6 out]
            }
            frame Enabled {
            }
          }
          n85 = call "IMAQ Particle Analysis"("Pixel Measurements"=w223, "Image"=w219) -> ("Particle Measurements (Pixels)"=w220:dbl[][])  [unwired: 3 in, 6 out]
          n86 = call "IMAQ Particle Analysis"("Pixel Measurements"=w218, "Image"=w219) -> ("Particle Measurements (Pixels)"=w217:dbl[][])  [unwired: 3 in, 6 out]
        }
        n87 = for {
          tunnel: w193 -> [w216] mode=indexing
          tunnel: [w215] -> w196 mode=indexing
          n88 = Index Array(array=w216) -> (element=w215:dbl[])  [unwired: 2 in]
        }
        n89 = for {
          tunnel: w194 -> [w212] mode=indexing
          tunnel: [w211] -> w195 mode=indexing
          n90 = Index Array(array=w212) -> (element=w211:dbl[])  [unwired: 2 in]
        }
        n91 = for {
          tunnel: w196 -> [w214] mode=indexing
          tunnel: [w213] -> w192 mode=indexing
          n92 = Index Array(array=w214) -> (element=w213:dbl)  [unwired: 1 in]
        }
        "粒长" <- w192
        n93 = for {
          tunnel: w195 -> [w210] mode=indexing
          tunnel: [w209] -> w191 mode=indexing
          n94 = Index Array(array=w210) -> (element=w209:dbl)  [unwired: 1 in]
        }
        "粒宽" <- w191
        n95 = call <vilib>:"Std Deviation and Variance.vi"("X"=w192) -> ("mean"=w189:dbl, "standard deviation"=w188:dbl)  [unwired: 1 in, 1 out]
        "mean 2" <- w189
        "standard deviation 2" <- w188
        n96 = call <vilib>:"Std Deviation and Variance.vi"("X"=w191) -> ("mean"=w187:dbl, "standard deviation"=w186:dbl)  [unwired: 1 in, 1 out]
        "mean 3" <- w187
        "standard deviation 3" <- w186
        n97 = Divide(x=w192, y=w191) -> (x/y=w190:dbl[])
        "长宽比" <- w190
        n98 = call <vilib>:"Std Deviation and Variance.vi"("X"=w190) -> ("mean"=w185:dbl, "standard deviation"=w184:dbl)  [unwired: 1 in, 1 out]
        "mean 4" <- w185
        "standard deviation 4" <- w184
      }
      frame #2 {
        n99 = Tick Count (ms)() -> (millisecond timer value=w280:u32)
        n100 = Subtract(x=w280, y=w279) -> (x-y=→"耗时":u32)
      }
    }
    n101 = Concatenate Strings(w25, ".png" ("string")) -> (w29:string)
    n102 = Build Path(base path="图片存储", name or relative path=w29) -> (appended path=w28:path)
    n103 = call-poly "IMAQ Write File 2"("File Path"=w28, "Image"=w24) -> ()  [unwired: 4 in, 6 out]
    n104 = call "IMAQ Particle Analysis"("Pixel Measurements"=w79, "Image"=w6) -> ("Particle Measurements (Pixels)"=w73:dbl[][])  [unwired: 3 in, 6 out]
    n105 = Index Array(array=w73, index (col)=0 ("index (row)")) -> (element=w72:dbl[])  [unwired: 1 in]
    "Area" <- w72
    n106 = Index Array(array=w73, index (col)=1 ("index (row)")) -> (element=w71:dbl[])  [unwired: 1 in]
    "Perimeter" <- w71
    n107 = Index Array(array=w73, index (col)=2 ("index (row)")) -> (element=w70:dbl[])  [unwired: 1 in]
    "AR" <- w70
    n108 = Index Array(array=w73, index (col)=3 ("index (row)")) -> (element=w69:dbl[])  [unwired: 1 in]
    "Equivalent ellipse" <- w69
    n109 = Index Array(array=w73, index (col)=4 ("index (row)")) -> (element=w68:dbl[])  [unwired: 1 in]
    "Circularity" <- w68
    n110 = call <vilib>:"Std Deviation and Variance.vi"("X"=w72) -> ("mean"=w59:dbl, "standard deviation"=w58:dbl)  [unwired: 1 in, 1 out]
    "mean 5" <- w59
    "standard deviation 5" <- w58
    n111 = call <vilib>:"Std Deviation and Variance.vi"("X"=w70) -> ("mean"=w55:dbl, "standard deviation"=w54:dbl)  [unwired: 1 in, 1 out]
    "mean 7" <- w55
    "standard deviation 7" <- w54
    n112 = call <vilib>:"Std Deviation and Variance.vi"("X"=w69) -> ("mean"=w53:dbl, "standard deviation"=w52:dbl)  [unwired: 1 in, 1 out]
    "mean 8" <- w53
    "standard deviation 8" <- w52
    n113 = call <vilib>:"Std Deviation and Variance.vi"("X"=w71) -> ("mean"=w57:dbl, "standard deviation"=w56:dbl)  [unwired: 1 in, 1 out]
    "mean 6" <- w57
    "standard deviation 6" <- w56
    n114 = call <vilib>:"Std Deviation and Variance.vi"("X"=w68) -> ("mean"=w51:dbl, "standard deviation"=w50:dbl)  [unwired: 1 in, 1 out]
    "mean 9" <- w51
    "standard deviation 9" <- w50
    n115 = Build Array(w67, w66, w65, w64, w63, w62, w59, w58, w57, w56, w55, w54, w53, w52, w51, w50) -> (w61:dbl[])
    n116 = Number To Fractional String(number=w61) -> (F-format string=w60:string[])  [unwired: 3 in]
    n117 = Build Array (concatenate)(w25, w47, w60) -> (w82:string[])
    n118 = call-poly <vilib>:"Write Delimited Spreadsheet.vi"("file path (dialog if empty)"="数据存储", "format (%s)"="%s", "1D data"=w82, "append to file? (new file:F)"=TRUE ("append to file? (F)")) -> ()  [unwired: 10 in, 2 out]
  }
